vi "加标回收数据插入.vi"(0 "data":T1={"时间"=timestamp(0 s since 1904-01-01), "参数"="水样测试", "数据类型"="N", "加标回收率"=0.0, "加标前水样测试时间"=timestamp(0 s since 1904-01-01), "加标前水样浓度值"=0.0, "加标后水样浓度值"=0.0, "加标母液浓度值"=0.0, "加标体积"=0.0, "加标水杯定容体积"=0.0}, 3 "错误输入（无错误）":errorcluster) -> (10 "错误输出":errorcluster)   [LabVIEW 2016]
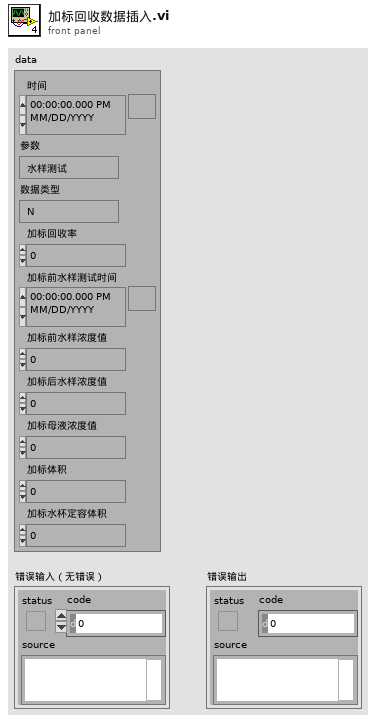
[diagram p1: front panel]
types:
  T1 = typedef "加标回收字段定义.ctl" = cluster{"时间":timestamp, "参数":string, "数据类型":string, "加标回收率":sgl, "加标前水样测试时间":timestamp, "加标前水样浓度值":sgl, "加标后水样浓度值":sgl, "加标母液浓度值":sgl, "加标体积":sgl, "加标水杯定容体积":sgl}
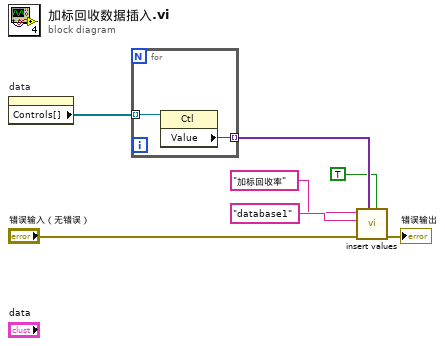
[diagram p0: block diagram]
diagram:
  n1 = property on="data" class="Clust (严格)"() -> ("Controls[]"=w7:refnum<vi>[])  [unwired: 2 in, 2 out]
  n2 = for {
    tunnel: w7 -> [w9] mode=indexing
    tunnel: [w8] -> w6 mode=indexing
    n3 = property class="Ctl"(reference=w9) -> ("Value"=w8:variant)  [unwired: 1 in, 2 out]
  }
  n4 = call "insert values.vi"("是否创建唯一键"=TRUE, "data"=w6, "错误输入（无错误）"="错误输入（无错误）", "database"="database1", "Tabe Name"="加标回收率") -> ("错误输出"=→"错误输出":errorcluster)  [unwired: 6 in]
